vi "Router - Get Imported Ch Indexes and Block Sizes.vi"(8 "error in (no error)":errorcluster, 11 "Imported Channel List":string[](array[string])) -> (0 "error out":errorcluster, 2 "Block Sizes":i32[](array[numeric]), 3 "Indexes":i32[](array[numeric]))   [LabVIEW 2016]
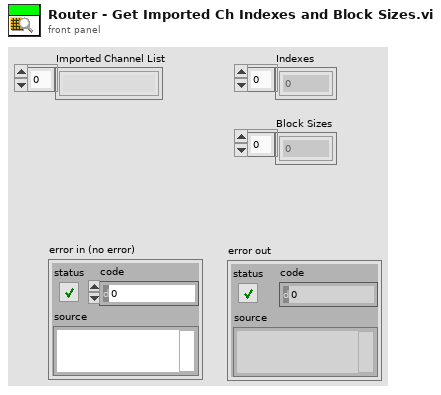
[diagram p1: front panel]
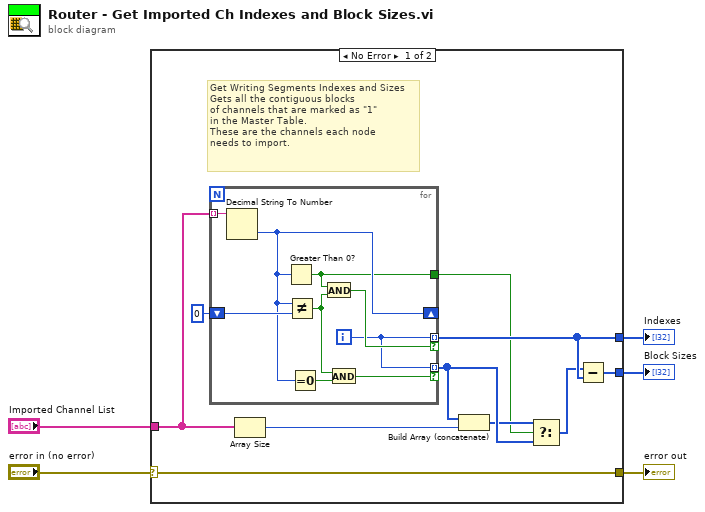
[diagram p0: block diagram]
diagram:
  n1 = case shown="No Error" "error in (no error)" {
    selector: "error in (no error)" -> [w6 w25]
    tunnel: "Imported Channel List" -> [w15 _]
    tunnel: [w14 _] -> w4
    tunnel: [w13 _] -> w3
    tunnel: [w6 w25] -> w1
    frame No Error {
      # "Get Writing Segments Indexes and Sizes\nGets all the contiguous blocks\nof channels that are marked as \"1\"\nin the Master Table.\nThese are the channels each node \nneeds to import."
      n2 = for {
        tunnel: w15 -> [w24] mode=indexing
        shift-right: [w19] -> _
        shift-left: 0 -> [w23]
        tunnel: [w18] -> w13 mode=indexing if=w22
        tunnel: [w18] -> w11 mode=indexing if=w17
        tunnel: [w16] -> w9
        i -> [w18]
        n3 = Decimal String To Number(string=w24) -> (number=w19:i32)  [unwired: 2 in, 1 out]
        n4 = Greater Than 0?(x=w19) -> (x > 0?=w16:bool)
        n5 = Not Equal?(x=w19, y=w23) -> (x != y?=w20:bool)
        n6 = Equal To 0?(x=w19) -> (x = 0?=w21:bool)
        n7 = And(x=w16, y=w20) -> (x .and. y?=w22:bool)
        n8 = And(x=w20, y=w21) -> (x .and. y?=w17:bool)
      }
      n9 = Array Size(array=w15) -> (size(s)=w8:i32)
      n10 = Build Array (concatenate)(w11, w8) -> (w10:i32[])
      n11 = Select(t=w10, s=w9, f=w11) -> (s? t:f=w12:i32[])
      n12 = Subtract(x=w12, y=w13) -> (x-y=w14:i32[])
    }
    frame Error {
    }
  }
  "Block Sizes" <- w4
  "Indexes" <- w3
  "error out" <- w1
